vi "GetBLFindDllPath.vi"(8 "error in (no error)":errorcluster, 11 "DLL Path":path) -> (0 "error out":errorcluster, 3 "BlfindDLLPath":path)   [LabVIEW 2022 SP3, in "EClib functions.lvlib"]
uses:
  EClib functions.lvlib
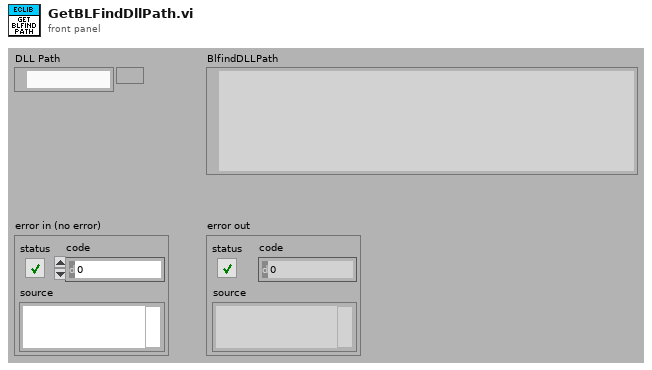
[diagram p1: front panel]
types:
  T1 = enum32{"invalid app kind", "Development System", "Run Time System", "Student Edition", "Embedded LabVIEW", "Evaluation", "Custom"}
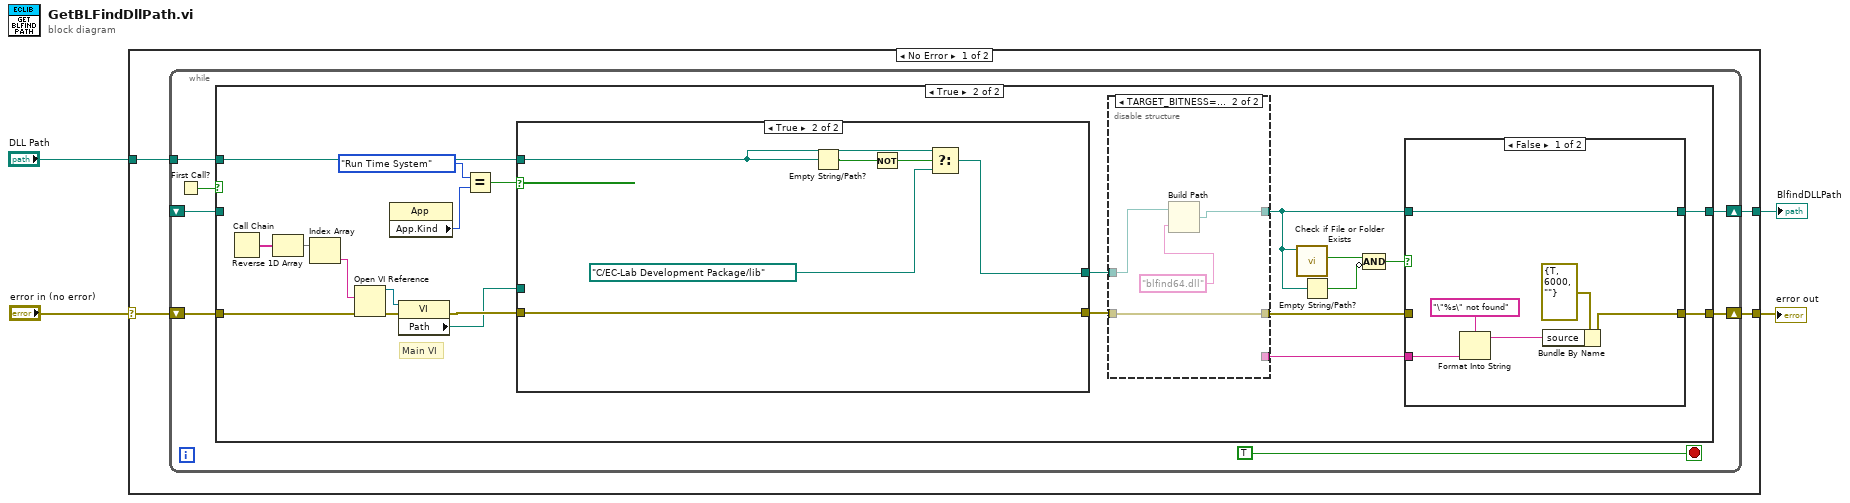
[diagram p0: block diagram]
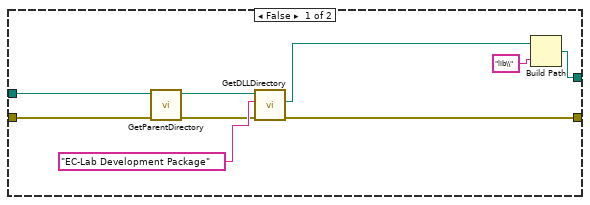
[diagram p3: hidden frame]
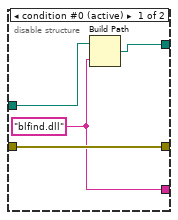
[diagram p5: hidden frame]
diagram:
  n1 = case shown="No Error" "error in (no error)" {
    selector: "error in (no error)" -> [w7 w71]
    tunnel: [w8 _] -> w4
    tunnel: [w6 w71] -> w2
    tunnel: "DLL Path" -> [w5 _]
    frame No Error {
      n2 = while {
        shift-right: [w13] -> w6
        shift-left: w7 -> [w14]
        shift-right: [w15] -> w8
        shift-left: _ -> [w10]
        tunnel: w5 -> [w9]
        stop <- TRUE stop-if-true
        n3 = First Call?() -> (First Call?: T/F=w11:bool)
        n4 = case shown="True" w11 {
          tunnel: [w17 w27] -> w15
          tunnel: w14 -> [w16 w34]
          tunnel: [w16 w30] -> w13
          tunnel: w10 -> [w17 _]
          tunnel: w9 -> [_ w18]
          frame False {
          }
          frame True {
            # "Main VI"
            n5 = Call Chain() -> (call chain=w36:string[])
            n6 = Reverse 1D Array(array=w36) -> (reversed array=w35:string[])
            n7 = Index Array(array=w35) -> (element=w37:string)  [unwired: 1 in]
            n8 = Open VI Reference(vi path=w37, error in (no error)=w34) -> (vi reference=w39:refnum<vi>, error out=w38:errorcluster)  [unwired: 4 out]
            n9 = property class="App"() -> ("App.Kind"=w24:T1)  [unwired: 2 in, 2 out]
            n10 = property class="VI"(reference=w39, error in=w38) -> (error out=w20:errorcluster, "Path"=w19:path)  [unwired: 1 out]
            n11 = Equal?(x=T1."Run Time System" ("Application:Kind"), y=w24) -> (x = y?=w23:bool)
            n12 = case shown="True" w23 {
              tunnel: [w46 w54] -> w22
              tunnel: [w47 w49] -> w21
              tunnel: w20 -> [w43 w54]
              tunnel: w19 -> [w42 _]
              tunnel: w18 -> [_ w51]
              frame False {
                n13 = call "GetParentDirectory.vi"("error in"=w43, "VIPath"=w42) -> ("error out"=w41:errorcluster, "VIRelativePath"=w40:path)  [unwired: 7 in, 1 out]
                n14 = call "GetDLLDirectory.vi"("error in (no error)"=w41, "DLLDirectoryName"="EC-Lab Development Package", "AppParentDirectory"=w40) -> ("error out"=w46:errorcluster, "DLLDirectory"=w45:path)  [unwired: 6 in, 1 out]
                n15 = Build Path(base path=w45, name or relative path="lib\\") -> (appended path=w47:path)
              }
              frame True {
                n16 = Empty String/Path?(string/path=w51) -> (empty?=w53:bool)
                n17 = Not(x=w53) -> (.not. x?=w52:bool)
                n18 = Select(t=w51, s=w52, f=path "C:/EC-Lab Development Package/lib" ("base path")) -> (s? t:f=w49:path)
              }
            }
            n19 = disable-structure shown="TARGET_BITNESS==64" {
              disable-tunnel: [w66 w70] -> w28
              disable-tunnel: w22 -> [w65 w69]
              disable-tunnel: [w65 w69] -> w31
              disable-tunnel: w21 -> [w63 w67]
              disable-tunnel: [w64 _] -> w26
              frame condition #0 (active) {
                w64 = "blfind.dll" ("name or relative path")
                n20 = Build Path(base path=w63, name or relative path=w64) -> (appended path=w66:path)
              }
              frame condition #1 {
                n21 = Build Path(base path=w67, name or relative path="blfind64.dll") -> (appended path=w70:path)
              }
            }
            n22 = call <vilib>:"Check if File or Folder Exists.vi"("path"=w28) -> ("file or folder exists?"=w33:bool)  [unwired: 8 in, 2 out]
            n23 = Empty String/Path?(string/path=w28) -> (empty?=w32:bool)
            n24 = Compound Arithmetic op=AND(w33, invert w32) -> (w29:bool)
            n25 = case shown="False" w29 {
              tunnel: w31 -> [_ w62]
              tunnel: [w58 w62] -> w30
              tunnel: w28 -> [w60 w61]
              tunnel: [w60 w61] -> w27
              tunnel: w26 -> [w57 _]
              frame False {
                n26 = Format Into String(format string="\"%s\" not found", w57) -> (resulting string=w55:string)  [unwired: 2 in, 1 out]
                n27 = Bundle By Name(cluster=errorcluster {"status"=TRUE, "code"=6000, "source"=""} ("error out"), "source"=w55) -> (w58:errorcluster)
              }
              frame True {
              }
            }
          }
        }
      }
    }
    frame Error {
    }
  }
  "BlfindDLLPath" <- w4
  "error out" <- w2
